vi "img.average.vi"(8 "error in":errorcluster, 10 "Array in":u16[][][](array[numeric])) -> (0 "errorthru":errorcluster, 2 "Array out":dbl[][](array[numeric]))   [LabVIEW 2020]
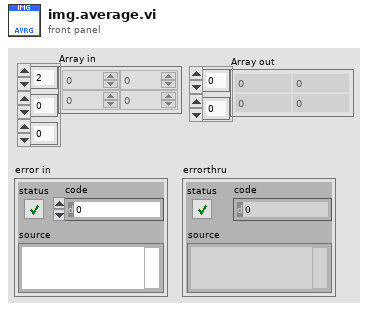
[diagram p1: front panel]
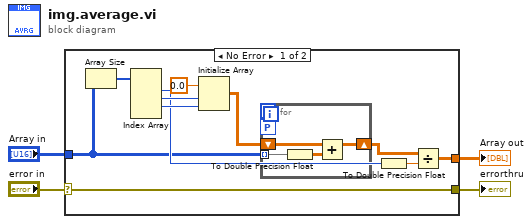
[diagram p0: block diagram]
diagram:
  n1 = case shown="No Error" "error in" {
    selector: "error in" -> [w7 w20]
    tunnel: "Array in" -> [w8 _]
    tunnel: [w9 _] -> w3
    tunnel: [w7 w20] -> w1
    frame No Error {
      n2 = Array Size(array=w8) -> (size(s)=w13:i32[])
      n3 = Index Array(array=w13) -> (element #1=w10:i32, element #2=w11:i32, element #3=w12:i32)  [unwired: 4 in, 1 out]
      n4 = Initialize Array(0.0, w11, w12) -> (w14:dbl[][])
      n5 = for {
        tunnel: w8 -> [w17] mode=indexing
        shift-right: [w18] -> w5
        shift-left: w14 -> [w19]
        workers-P: _ -> [_]
        n6 = To Double Precision Float(number=w17) -> (double precision float=w16:dbl[][])
        n7 = Add(x=w19, y=w16) -> (x+y=w18:dbl[][])
      }
      n8 = To Double Precision Float(number=w10) -> (double precision float=w6:dbl)
      n9 = Divide(x=w5, y=w6) -> (x/y=w9:dbl[][])
    }
    frame Error {
    }
  }
  "Array out" <- w3
  "errorthru" <- w1
